vi "Init VI.vi"(8 "error in (no error)":errorcluster, 11 "VI in":refnum<vi>) -> (0 "error out":errorcluster)   [LabVIEW 2018]
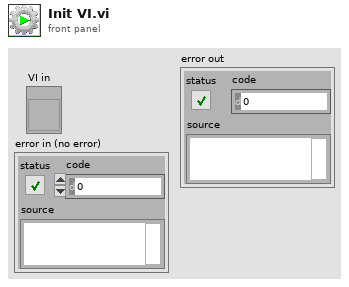
[diagram p1: front panel]
types:
  T1 = enum32{"Invalid", "Standard", "Closed", "Hidden", "Minimized", "Maximized"}
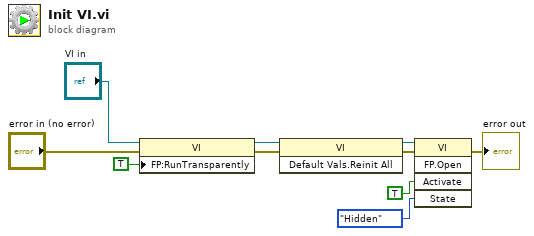
[diagram p0: block diagram]
diagram:
  n1 = property class="VI"(reference="VI in", error in="error in (no error)", "FP:RunTransparently"=TRUE ("Front Panel Window:Run VI Transparently")) -> (reference out=w1:refnum<vi>, error out=w2:errorcluster)
  n2 = invoke class="VI" method="Default Vals.Reinit All"(reference=w1, error in=w2) -> (reference out=w4:refnum<vi>, error out=w3:errorcluster)  [unwired: 1 in, 1 out]
  n3 = invoke class="VI" method="FP.Open"(reference=w4, error in=w3, "Activate"=TRUE ("Activate?"), "State"=T1."Hidden") -> (error out=→"error out":errorcluster)  [unwired: 1 in, 4 out]
